vi "Ball Shooter Tasks.vi"(0 "Ball Shooter Task Parameters":T1) -> ()   [LabVIEW 2015]
uses:
  <vilib>/Rock Robotics/WPI/Relay/WPI_RelayValue.ctl
  Robot Global Data.vi
  <vilib>/Rock Robotics/Network Tables/NT Write Number.vi
  <vilib>/Rock Robotics/WPI/Utilities/WPI_GetSetVariantRefNum.vi
  <vilib>/Rock Robotics/Network Tables/NT Read Boolean.vi
  <vilib>/Rock Robotics/WPI/RobotDrive/WPI_RobotDriveArcadeDrive_Standard(NoSaturation).vi
  <vilib>/Rock Robotics/Network Tables/NT Write Numeric Array.vi
  <vilib>/Rock Robotics/Network Tables/NT Read Number.vi
panel:
  out "Shooter Lift Motor":dbl
  out "Drive Motor Values":dbl[](array[numeric])
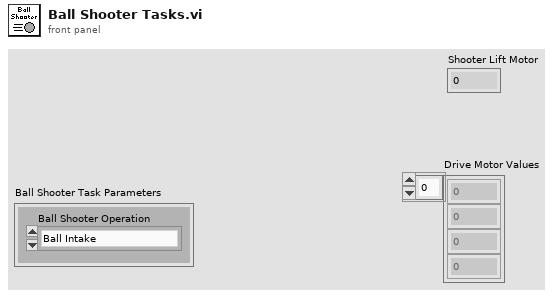
[diagram p1: front panel]
types:
  T1 = cluster{"Ball Shooter Operation":enum16{"Ball Intake", "Fire Ball Shooter", "Aim Ball Shooter"}}
  T2 = typedef "WPI_RelayValue.ctl" = enum16{"Off", "On", "Forward", "Reverse"}
  T3 = enum16{"Ball Intake", "Fire Ball Shooter", "Aim Ball Shooter"}
  T4 = typedef "WPI_MotorControlDeviceRef.ctl" = cluster{"DeviceStatus":errorcluster, "Type":T5, "PWM":cluster{"PWM Channel":T6, "DeadBand":T7}, "CAN":cluster{"Device Number":u8, "Control Mode":T8, "Semaphore":T9, "Max Vout":dbl, "TalonSRX Control Mode":T10}, "Invert":bool}
  T5 = typedef "WPI_MotorControlType.ctl" = enum16{"PWM", "CAN", "CANTalonSRX"}
  T6 = typedef "FPGA_DIOPWMChannel.ctl" = enum8{"PWM 0", "PWM 1", "PWM 2", "PWM 3", "PWM 4", "PWM 5", "PWM 6", "PWM 7", "PWM 8", "PWM 9", "PWM MXP 0", "PWM MXP 1", "PWM MXP 2", "PWM MXP 3", "PWM MXP 4", "PWM MXP 5", "PWM MXP 6", "PWM MXP 7", "PWM MXP 8", "PWM MXP 9", "Invalid"}
  T7 = typedef "WPI_PWMDeadband.ctl" = cluster{"Name":string, "maxPositivePwm":i32, "minPositivePwm":i32, "centerPwm":i32, "maxNegativePwm":i32, "minNegativePwm":i32, "angularRange":u16}
  T8 = typedef "WPI_CANJaguar_ControlMode.ctl" = enum8{"Percent VBus", "Current", "Speed", "Position", "Voltage"}
  T9 = typedef "Semaphore RefNum" = refnum<k1>
  T10 = typedef "WPI_CANTalonSRX_APIControlMode.ctl" = enum8{"Percent VBus", "Speed", "Position", "Slave", "Unchanged / Invalid", "Voltage Compensation", "Current", "Motion Profile"}
  T11 = typedef "WPI_RelayDevRef.ctl" = cluster{"DevStatus":errorcluster, "Relay Channel":T12, "Relay Direction":T13}
  T12 = typedef "FPGA_DIORelayChannel.ctl" = enum8{"Relay 0", "Relay 1", "Relay 2", "Relay 3", "Invalid"}
  T13 = typedef "WPI_RelayDirection.ctl" = enum16{"Both directions", "Forward only", "Reverse only"}
  T14 = typedef "WPI_RobotDriveDevRef.ctl" = cluster{"DevStatus":errorcluster, "Motors[]":T4[], "Square Inputs":bool, "Max Output":dbl}
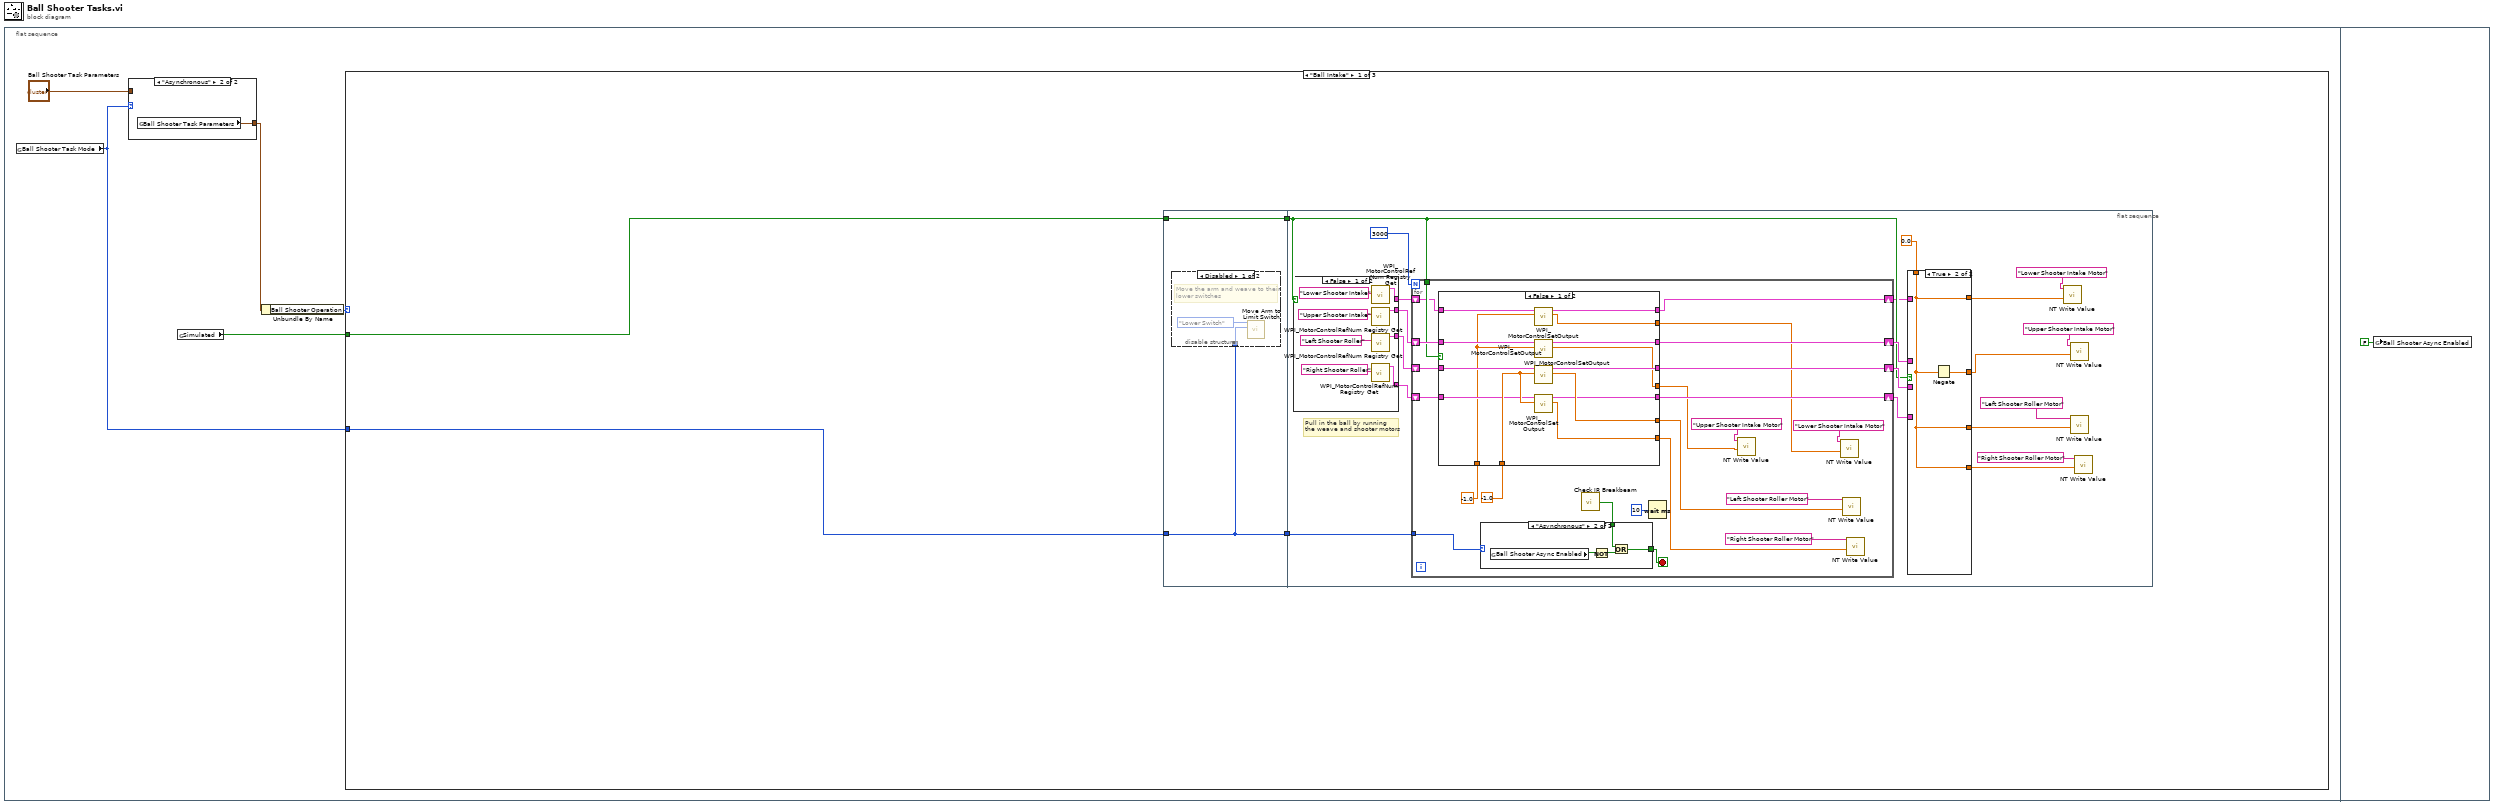
[diagram p0: block diagram]
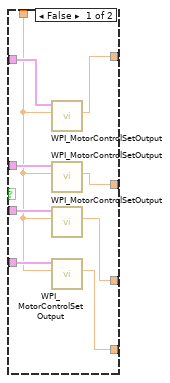
[diagram p4: hidden frame]
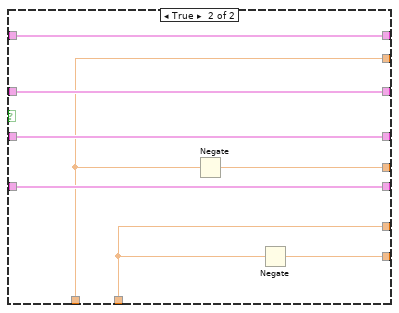
[diagram p5: hidden frame]
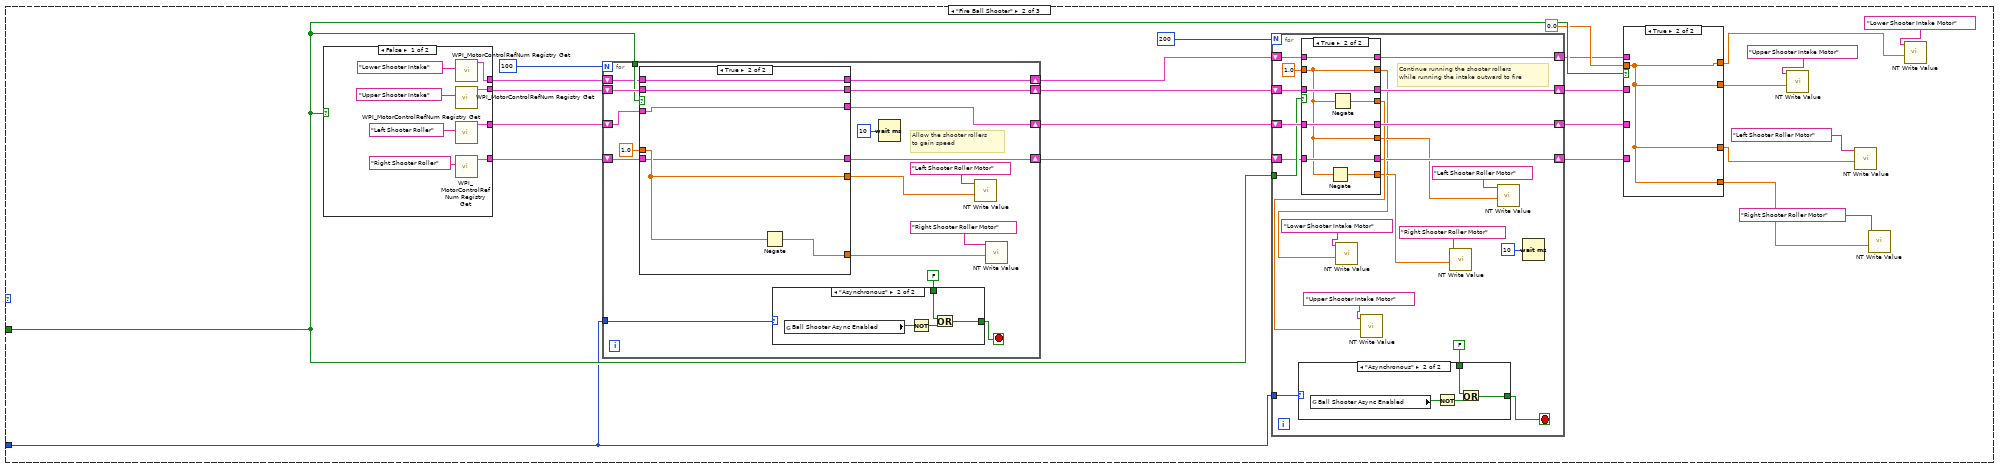
[diagram p7: hidden frame]
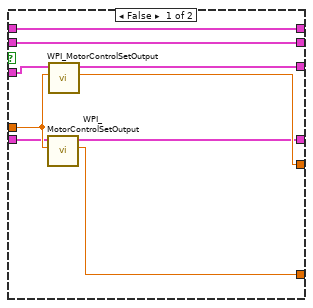
[diagram p8: hidden frame]
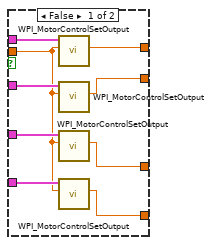
[diagram p10: hidden frame]
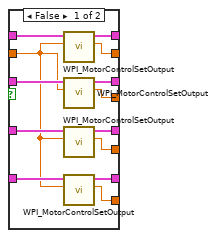
[diagram p12: hidden frame]
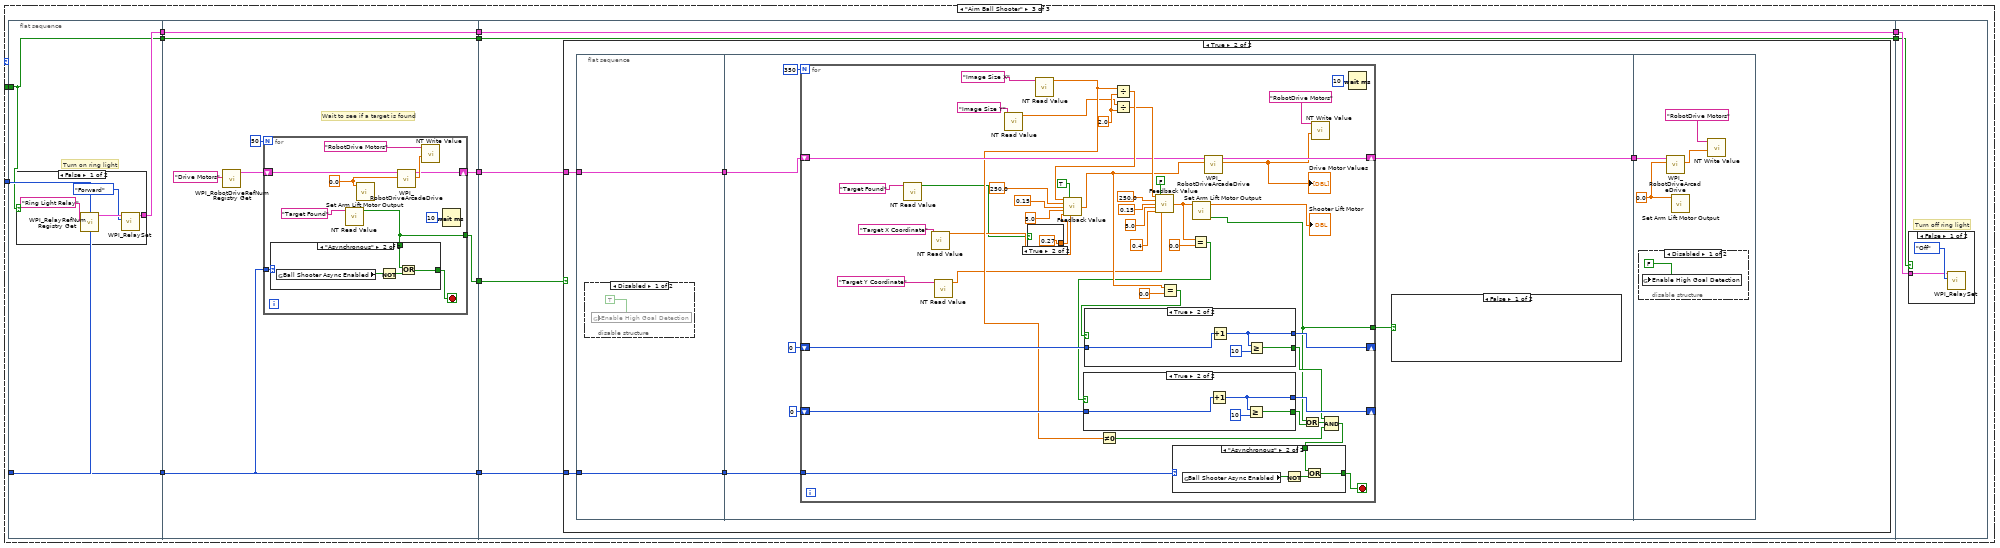
[diagram p14: hidden frame]
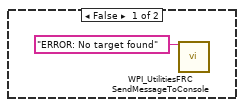
[diagram p17: hidden frame]
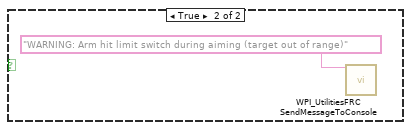
[diagram p19: hidden frame]
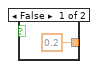
[diagram p20: hidden frame]
diagram:
  n1 = flat-sequence {
    frame #0 {
      n2 = global read "Robot Global Data.vi" "Ball Shooter Task Mode"() -> (w3:enum16{"Synchronous", "Asynchronous"})
      n3 = case shown="\"Asynchronous\"" w3 {
        tunnel: [w370 w371] -> w5
        tunnel: "Ball Shooter Task Parameters" -> [w370 _]
        frame "Synchronous" {
        }
        frame "Asynchronous" {
          n4 = global read "Robot Global Data.vi" "Ball Shooter Task Parameters"() -> (w371:T1)
        }
      }
      n5 = global read "Robot Global Data.vi" "Simulated"() -> (w1:bool)
      n6 = Unbundle By Name(w5) -> ("Ball Shooter Operation"=w4:T3)
      n7 = case shown="\"Ball Intake\"" w4 {
        tunnel: w3 -> [w8 w118 w242]
        tunnel: w1 -> [w9 w119 w235]
        frame "Ball Intake" {
          n8 = flat-sequence {
            tunnel: w8 -> [w10]
            tunnel: w9 -> [w11]
            tunnel: [w11] -> w7
            tunnel: [w10] -> w6
            tunnel: w7 -> [w27]
            tunnel: w6 -> [w30]
            frame #0 {
              n9 = disable-structure shown="Disabled" {
                disable-tunnel: w10 -> [w12 _]
                frame Disabled {
                  # "Move the arm and weave to their\nlower switches"
                  n10 = call "Move Arm to Limit Switch.vi"("Call Mode"=w12, "Switch"=enum16{"Lower Switch", "Upper Switch"}."Lower Switch") -> ()  [unwired: 10 in]
                }
                frame Enabled {
                }
              }
            }
            frame #1 {
              # "Pull in the ball by running\nthe weave and shooter motors"
              n11 = case shown="False" w27 {
                tunnel: [w41 _] -> w29
                tunnel: [w39 _] -> w28
                tunnel: [w36 _] -> w26
                tunnel: [w34 _] -> w19
                frame False {
                  n12 = call <vilib>:"WPI_MotorControlRefNum Registry Get.vi"("refnum name"="Upper Shooter Intake") -> ("MotorControlDevRef"=w39:T4)  [unwired: 9 in, 1 out]
                  n13 = call <vilib>:"WPI_MotorControlRefNum Registry Get.vi"("refnum name"="Left Shooter Roller") -> ("MotorControlDevRef"=w41:T4)  [unwired: 9 in, 1 out]
                  n14 = call <vilib>:"WPI_MotorControlRefNum Registry Get.vi"("refnum name"="Right Shooter Roller") -> ("MotorControlDevRef"=w36:T4)  [unwired: 9 in, 1 out]
                  n15 = call <vilib>:"WPI_MotorControlRefNum Registry Get.vi"("refnum name"="Lower Shooter Intake") -> ("MotorControlDevRef"=w34:T4)  [unwired: 9 in, 1 out]
                }
                frame True {
                }
              }
              n16 = for {
                N: 3000 -> [_]
                tunnel: w30 -> [w75]
                shift-right: [w71] -> w31
                shift-left: w28 -> [w72]
                shift-right: [w69] -> w32
                shift-left: w29 -> [w70]
                tunnel: w27 -> [w68]
                shift-right: [w60] -> w25
                shift-left: w26 -> [w61]
                shift-right: [w56] -> w18
                shift-left: w19 -> [w57]
                stop <- w74 stop-if-true
                n17 = case shown="False" w68 {
                  tunnel: w72 -> [w89 w97]
                  tunnel: [w88 w97] -> w71
                  tunnel: w70 -> [w87 w96]
                  tunnel: [w86 w96] -> w69
                  tunnel: [w85 w91] -> w54
                  tunnel: [w84 w93] -> w65
                  tunnel: -1.0 -> [w83 w93]
                  tunnel: -1.0 -> [w77 w90]
                  tunnel: w61 -> [w82 w95]
                  tunnel: [w81 w95] -> w60
                  tunnel: [w80 w94] -> w58
                  tunnel: w57 -> [w79 w92]
                  tunnel: [w78 w92] -> w56
                  tunnel: [w76 w90] -> w53
                  frame False {
                    n18 = call <vilib>:"WPI_MotorControlSetOutput.vi"("Output"=w77, "MotorControlDevRef"=w79) -> ("Motor Output"=w76:dbl, "MotorControlDevRef"=w78:T4)  [unwired: 7 in, 1 out]
                    n19 = call <vilib>:"WPI_MotorControlSetOutput.vi"("Output"=w77, "MotorControlDevRef"=w89) -> ("Motor Output"=w85:dbl, "MotorControlDevRef"=w88:T4)  [unwired: 7 in, 1 out]
                    n20 = call <vilib>:"WPI_MotorControlSetOutput.vi"("Output"=w83, "MotorControlDevRef"=w87) -> ("Motor Output"=w84:dbl, "MotorControlDevRef"=w86:T4)  [unwired: 7 in, 1 out]
                    n21 = call <vilib>:"WPI_MotorControlSetOutput.vi"("Output"=w83, "MotorControlDevRef"=w82) -> ("Motor Output"=w80:dbl, "MotorControlDevRef"=w81:T4)  [unwired: 7 in, 1 out]
                  }
                  frame True {
                    n22 = Negate(x=w90) -> (-x=w91:dbl)
                    n23 = Negate(x=w93) -> (-x=w94:dbl)
                  }
                }
                n24 = call "Check IR Breakbeam.vi"() -> ("Beam Broken"=w67:bool)
                n25 = case shown="\"Asynchronous\"" w75 {
                  tunnel: [w98 w100] -> w74
                  tunnel: w67 -> [w98 w99]
                  frame "Synchronous" {
                  }
                  frame "Asynchronous" {
                    n26 = global read "Robot Global Data.vi" "Ball Shooter Async Enabled"() -> (w101:bool)
                    n27 = Not(x=w101) -> (.not. x?=w102:bool)
                    n28 = Or(x=w99, y=w102) -> (x .or. y?=w100:bool)
                  }
                }
                n29 = Wait (ms)(milliseconds to wait=u32 10) -> ()  [unwired: 1 out]
                n30 = call-poly <vilib>:"NT Write Value.vi"("Numeric"=w54, "Name"="Upper Shooter Intake Motor" ("refnum name")) -> ()  [unwired: 9 in, 1 out]
                n31 = call-poly <vilib>:"NT Write Value.vi"("Numeric"=w53, "Name"="Lower Shooter Intake Motor" ("refnum name")) -> ()  [unwired: 9 in, 1 out]
                n32 = call-poly <vilib>:"NT Write Value.vi"("Numeric"=w65, "Name"="Left Shooter Roller Motor" ("refnum name")) -> ()  [unwired: 9 in, 1 out]
                n33 = call-poly <vilib>:"NT Write Value.vi"("Numeric"=w58, "Name"="Right Shooter Roller Motor" ("refnum name")) -> ()  [unwired: 9 in, 1 out]
              }
              n34 = case shown="True" w27 {
                tunnel: w32 -> [w50 _]
                tunnel: w31 -> [w49 _]
                tunnel: w25 -> [w48 _]
                tunnel: [w47 w52] -> w14
                tunnel: [w46 w51] -> w22
                tunnel: [w45 w51] -> w21
                tunnel: 0.0 -> [w43 w51]
                tunnel: w18 -> [w44 _]
                tunnel: [w42 w51] -> w15
                frame False {
                  n35 = call <vilib>:"WPI_MotorControlSetOutput.vi"("Output"=w43, "MotorControlDevRef"=w44) -> ("Motor Output"=w42:dbl)  [unwired: 7 in, 2 out]
                  n36 = call <vilib>:"WPI_MotorControlSetOutput.vi"("Output"=w43, "MotorControlDevRef"=w49) -> ("Motor Output"=w47:dbl)  [unwired: 7 in, 2 out]
                  n37 = call <vilib>:"WPI_MotorControlSetOutput.vi"("Output"=w43, "MotorControlDevRef"=w50) -> ("Motor Output"=w46:dbl)  [unwired: 7 in, 2 out]
                  n38 = call <vilib>:"WPI_MotorControlSetOutput.vi"("Output"=w43, "MotorControlDevRef"=w48) -> ("Motor Output"=w45:dbl)  [unwired: 7 in, 2 out]
                }
                frame True {
                  n39 = Negate(x=w51) -> (-x=w52:dbl)
                }
              }
              n40 = call-poly <vilib>:"NT Write Value.vi"("Numeric"=w15, "Name"="Lower Shooter Intake Motor" ("refnum name")) -> ()  [unwired: 9 in, 1 out]
              n41 = call-poly <vilib>:"NT Write Value.vi"("Numeric"=w14, "Name"="Upper Shooter Intake Motor" ("refnum name")) -> ()  [unwired: 9 in, 1 out]
              n42 = call-poly <vilib>:"NT Write Value.vi"("Numeric"=w22, "Name"="Left Shooter Roller Motor" ("refnum name")) -> ()  [unwired: 9 in, 1 out]
              n43 = call-poly <vilib>:"NT Write Value.vi"("Numeric"=w21, "Name"="Right Shooter Roller Motor" ("refnum name")) -> ()  [unwired: 9 in, 1 out]
            }
          }
        }
        frame "Fire Ball Shooter" {
          n44 = case shown="False" w119 {
            tunnel: [w182 _] -> w123
            tunnel: [w179 _] -> w122
            tunnel: [w178 _] -> w114
            tunnel: [w176 _] -> w107
            frame False {
              n45 = call <vilib>:"WPI_MotorControlRefNum Registry Get.vi"("refnum name"="Upper Shooter Intake") -> ("MotorControlDevRef"=w182:T4)  [unwired: 9 in, 1 out]
              n46 = call <vilib>:"WPI_MotorControlRefNum Registry Get.vi"("refnum name"="Left Shooter Roller") -> ("MotorControlDevRef"=w179:T4)  [unwired: 9 in, 1 out]
              n47 = call <vilib>:"WPI_MotorControlRefNum Registry Get.vi"("refnum name"="Right Shooter Roller") -> ("MotorControlDevRef"=w178:T4)  [unwired: 9 in, 1 out]
              n48 = call <vilib>:"WPI_MotorControlRefNum Registry Get.vi"("refnum name"="Lower Shooter Intake") -> ("MotorControlDevRef"=w176:T4)  [unwired: 9 in, 1 out]
            }
            frame True {
            }
          }
          n49 = for {
            N: 100 -> [_]
            shift-right: [w139] -> w121
            shift-left: w122 -> [w140]
            shift-right: [w142] -> w120
            shift-left: w123 -> [w141]
            tunnel: w119 -> [w138]
            tunnel: w118 -> [w137]
            shift-right: [w130] -> w113
            shift-left: w114 -> [w131]
            shift-right: [w128] -> w106
            shift-left: w107 -> [w129]
            stop <- w144 stop-if-true
            # "Allow the shooter rollers\nto gain speed"
            n50 = case shown="True" w138 {
              tunnel: [w154 w160] -> w142
              tunnel: w141 -> [w154 w160]
              tunnel: w140 -> [w153 w159]
              tunnel: [w152 w159] -> w139
              tunnel: 1.0 ("Output") -> [w151 w157]
              tunnel: [w150 w157] -> w133
              tunnel: [w149 w158] -> w132
              tunnel: w131 -> [w148 w156]
              tunnel: [w147 w156] -> w130
              tunnel: w129 -> [w146 w155]
              tunnel: [w146 w155] -> w128
              frame False {
                n51 = call <vilib>:"WPI_MotorControlSetOutput.vi"("Output"=w151, "MotorControlDevRef"=w148) -> ("Motor Output"=w149:dbl, "MotorControlDevRef"=w147:T4)  [unwired: 7 in, 1 out]
                n52 = call <vilib>:"WPI_MotorControlSetOutput.vi"("Output"=w151, "MotorControlDevRef"=w153) -> ("Motor Output"=w150:dbl, "MotorControlDevRef"=w152:T4)  [unwired: 7 in, 1 out]
              }
              frame True {
                n53 = Negate(x=w157) -> (-x=w158:dbl)
              }
            }
            n54 = case shown="\"Asynchronous\"" w137 {
              tunnel: FALSE -> [w161 w163]
              tunnel: [w161 w162] -> w144
              frame "Synchronous" {
              }
              frame "Asynchronous" {
                n55 = global read "Robot Global Data.vi" "Ball Shooter Async Enabled"() -> (w164:bool)
                n56 = Not(x=w164) -> (.not. x?=w165:bool)
                n57 = Or(x=w163, y=w165) -> (x .or. y?=w162:bool)
              }
            }
            n58 = Wait (ms)(milliseconds to wait=u32 10) -> ()  [unwired: 1 out]
            n59 = call-poly <vilib>:"NT Write Value.vi"("Numeric"=w133, "Name"="Left Shooter Roller Motor" ("refnum name")) -> ()  [unwired: 9 in, 1 out]
            n60 = call-poly <vilib>:"NT Write Value.vi"("Numeric"=w132, "Name"="Right Shooter Roller Motor" ("refnum name")) -> ()  [unwired: 9 in, 1 out]
          }
          n61 = for {
            N: 200 -> [_]
            shift-right: [w202] -> w127
            shift-left: w120 -> [w204]
            shift-right: [w201] -> w126
            shift-left: w121 -> [w203]
            tunnel: w118 -> [w199]
            tunnel: w119 -> [w197]
            shift-right: [w190] -> w112
            shift-left: w113 -> [w191]
            shift-right: [w186] -> w105
            shift-left: w106 -> [w187]
            stop <- w205 stop-if-true
            # "Continue running the shooter rollers\nwhile running the intake outward to fire"
            n62 = case shown="\"Asynchronous\"" w199 {
              tunnel: FALSE -> [w226 w228]
              tunnel: [w226 w227] -> w205
              frame "Synchronous" {
              }
              frame "Asynchronous" {
                n63 = global read "Robot Global Data.vi" "Ball Shooter Async Enabled"() -> (w229:bool)
                n64 = Not(x=w229) -> (.not. x?=w230:bool)
                n65 = Or(x=w228, y=w230) -> (x .or. y?=w227:bool)
              }
            }
            n66 = case shown="True" w197 {
              tunnel: w204 -> [w218 w225]
              tunnel: w203 -> [w217 w224]
              tunnel: [w216 w225] -> w202
              tunnel: [w215 w224] -> w201
              tunnel: [w214 w220] -> w195
              tunnel: [w213 w219] -> w189
              tunnel: 1.0 -> [w209 w219]
              tunnel: w191 -> [w212 w223]
              tunnel: [w211 w223] -> w190
              tunnel: [w210 w222] -> w188
              tunnel: w187 -> [w208 w221]
              tunnel: [w207 w221] -> w186
              tunnel: [w206 w219] -> w184
              frame False {
                n67 = call <vilib>:"WPI_MotorControlSetOutput.vi"("Output"=w209, "MotorControlDevRef"=w208) -> ("Motor Output"=w206:dbl, "MotorControlDevRef"=w207:T4)  [unwired: 7 in, 1 out]
                n68 = call <vilib>:"WPI_MotorControlSetOutput.vi"("Output"=w209, "MotorControlDevRef"=w218) -> ("Motor Output"=w214:dbl, "MotorControlDevRef"=w216:T4)  [unwired: 7 in, 1 out]
                n69 = call <vilib>:"WPI_MotorControlSetOutput.vi"("Output"=w209, "MotorControlDevRef"=w217) -> ("Motor Output"=w213:dbl, "MotorControlDevRef"=w215:T4)  [unwired: 7 in, 1 out]
                n70 = call <vilib>:"WPI_MotorControlSetOutput.vi"("Output"=w209, "MotorControlDevRef"=w212) -> ("Motor Output"=w210:dbl, "MotorControlDevRef"=w211:T4)  [unwired: 7 in, 1 out]
              }
              frame True {
                n71 = Negate(x=w219) -> (-x=w222:dbl)
                n72 = Negate(x=w219) -> (-x=w220:dbl)
              }
            }
            n73 = call-poly <vilib>:"NT Write Value.vi"("Numeric"=w184, "Name"="Lower Shooter Intake Motor" ("refnum name")) -> ()  [unwired: 9 in, 1 out]
            n74 = call-poly <vilib>:"NT Write Value.vi"("Numeric"=w195, "Name"="Upper Shooter Intake Motor" ("refnum name")) -> ()  [unwired: 9 in, 1 out]
            n75 = call-poly <vilib>:"NT Write Value.vi"("Numeric"=w188, "Name"="Right Shooter Roller Motor" ("refnum name")) -> ()  [unwired: 9 in, 1 out]
            n76 = call-poly <vilib>:"NT Write Value.vi"("Numeric"=w189, "Name"="Left Shooter Roller Motor" ("refnum name")) -> ()  [unwired: 9 in, 1 out]
            n77 = Wait (ms)(milliseconds to wait=u32 10) -> ()  [unwired: 1 out]
          }
          n78 = case shown="True" w119 {
            tunnel: w127 -> [w174 _]
            tunnel: w126 -> [w173 _]
            tunnel: 0.0 -> [w167 w175]
            tunnel: [w172 w175] -> w115
            tunnel: [w171 w175] -> w109
            tunnel: w112 -> [w170 _]
            tunnel: [w169 w175] -> w108
            tunnel: w105 -> [w168 _]
            tunnel: [w166 w175] -> w103
            frame False {
              n79 = call <vilib>:"WPI_MotorControlSetOutput.vi"("Output"=w167, "MotorControlDevRef"=w168) -> ("Motor Output"=w166:dbl)  [unwired: 7 in, 2 out]
              n80 = call <vilib>:"WPI_MotorControlSetOutput.vi"("Output"=w167, "MotorControlDevRef"=w174) -> ("Motor Output"=w172:dbl)  [unwired: 7 in, 2 out]
              n81 = call <vilib>:"WPI_MotorControlSetOutput.vi"("Output"=w167, "MotorControlDevRef"=w173) -> ("Motor Output"=w171:dbl)  [unwired: 7 in, 2 out]
              n82 = call <vilib>:"WPI_MotorControlSetOutput.vi"("Output"=w167, "MotorControlDevRef"=w170) -> ("Motor Output"=w169:dbl)  [unwired: 7 in, 2 out]
            }
            frame True {
            }
          }
          n83 = call-poly <vilib>:"NT Write Value.vi"("Numeric"=w115, "Name"="Upper Shooter Intake Motor" ("refnum name")) -> ()  [unwired: 9 in, 1 out]
          n84 = call-poly <vilib>:"NT Write Value.vi"("Numeric"=w109, "Name"="Left Shooter Roller Motor" ("refnum name")) -> ()  [unwired: 9 in, 1 out]
          n85 = call-poly <vilib>:"NT Write Value.vi"("Numeric"=w108, "Name"="Right Shooter Roller Motor" ("refnum name")) -> ()  [unwired: 9 in, 1 out]
          n86 = call-poly <vilib>:"NT Write Value.vi"("Numeric"=w103, "Name"="Lower Shooter Intake Motor" ("refnum name")) -> ()  [unwired: 9 in, 1 out]
        }
        frame "Aim Ball Shooter" {
          n87 = flat-sequence {
            tunnel: w242 -> [w245]
            tunnel: [w245] -> w241
            tunnel: [w244] -> w236
            tunnel: w235 -> [w243]
            tunnel: [w243] -> w232
            tunnel: w241 -> [w255]
            tunnel: [w255] -> w240
            tunnel: [w256] -> w239
            tunnel: [w254] -> w237
            tunnel: w236 -> [w254]
            tunnel: [w253] -> w233
            tunnel: w232 -> [w253]
            tunnel: [w250] -> w231
            tunnel: w240 -> [w277]
            tunnel: w239 -> [w276]
            tunnel: [w275] -> w238
            tunnel: w237 -> [w275]
            tunnel: [w274] -> w234
            tunnel: w233 -> [w274]
            tunnel: w231 -> [w273]
            tunnel: w238 -> [w367]
            tunnel: w234 -> [w366]
            frame #0 {
              # "Turn on ring light"
              n88 = case shown="False" w243 {
                tunnel: [w246 _] -> w244
                frame False {
                  n89 = call <vilib>:"WPI_RelayRefNum Registry Get.vi"("refnum name"="Ring Light Relay") -> ("RelayDevRef"=w248:T11)  [unwired: 9 in, 1 out]
                  n90 = call <vilib>:"WPI_RelaySet.vi"("RelayValue"=WPI_RelayValue."Forward", "RelayDevRef"=w248) -> ("RelayDevRef"=w246:T11)  [unwired: 8 in, 1 out]
                }
                frame True {
                }
              }
            }
            frame #1 {
              # "Wait to see if a target is found"
              n91 = call <vilib>:"WPI_RobotDriveRefNum Registry Get.vi"("refnum name"="Drive Motors") -> ("RobotDriveDevRef"=w251:T14)  [unwired: 9 in, 1 out]
              n92 = for {
                N: 50 -> [_]
                tunnel: [w264] -> w256
                tunnel: w255 -> [w263]
                shift-right: [w258] -> w250
                shift-left: w251 -> [w259]
                stop <- w266 stop-if-true
                w260 = 0.0
                n93 = call-poly <vilib>:"NT Read Value.vi"("Name"="Target Found") -> ("Boolean"=w264:bool)  [unwired: 9 in, 1 out]
                n94 = case shown="\"Asynchronous\"" w263 {
                  tunnel: [w268 w270] -> w266
                  tunnel: w264 -> [w268 w269]
                  frame "Synchronous" {
                  }
                  frame "Asynchronous" {
                    n95 = global read "Robot Global Data.vi" "Ball Shooter Async Enabled"() -> (w271:bool)
                    n96 = Not(x=w271) -> (.not. x?=w272:bool)
                    n97 = Or(x=w269, y=w272) -> (x .or. y?=w270:bool)
                  }
                }
                n98 = call "Set Arm Lift Motor Output.vi"("Output"=w260) -> ()  [unwired: 7 in, 4 out]
                n99 = call-poly <vilib>:"WPI_RobotDriveArcadeDrive.vi"("X axis value"=w260, "RobotDriveDevRef"=w259) -> ("Motor Values"=w262:dbl[], "RobotDriveDevRef"=w258:T14)  [unwired: 7 in, 1 out]
                n100 = call-poly <vilib>:"NT Write Value.vi"("Numeric Array"=w262, "Name"="RobotDrive Motors") -> ()  [unwired: 9 in, 1 out]
                n101 = Wait (ms)(milliseconds to wait=u32 10) -> ()  [unwired: 1 out]
              }
            }
            frame #2 {
              n102 = case shown="True" w276 {
                tunnel: w277 -> [_ w281]
                tunnel: w273 -> [_ w279]
                frame False {
                  n103 = call <vilib>:"WPI_UtilitiesFRC SendMessageToConsole.vi"("Message"="ERROR: No target found") -> ()  [unwired: 14 in, 1 out]
                }
                frame True {
                  n104 = flat-sequence {
                    tunnel: w281 -> [w285]
                    tunnel: [w285] -> w283
                    tunnel: [w284] -> w280
                    tunnel: w279 -> [w284]
                    tunnel: w283 -> [w292]
                    tunnel: [w288] -> w282
                    tunnel: w280 -> [w287]
                    tunnel: w282 -> [w362]
                    frame #0 {
                      n105 = disable-structure shown="Disabled" {
                        frame Disabled {
                          n106 = global write "Robot Global Data.vi" "Enable High Goal Detection"(TRUE ("Enable Vision")) -> ()
                        }
                        frame Enabled {
                        }
                      }
                    }
                    frame #1 {
                      n107 = for {
                        N: 350 -> [_]
                        shift-right: [w327] -> w288
                        shift-left: w287 -> [w328]
                        tunnel: w292 -> [w324]
                        shift-right: [w320] -> _
                        shift-left: 0 -> [w321]
                        shift-right: [w318] -> _
                        shift-left: 0 -> [w319]
                        tunnel: [w307] -> w289
                        stop <- w325 stop-if-true
                        w336 = 2.0
                        n108 = call-poly <vilib>:"NT Read Value.vi"("Name"="Target Found") -> ("Boolean"=w296:bool)  [unwired: 9 in, 1 out]
                        n109 = call-poly <vilib>:"NT Read Value.vi"("Name"="Target X Coordinate") -> ("Numeric"=w299:dbl)  [unwired: 9 in, 1 out]
                        n110 = call-poly <vilib>:"NT Read Value.vi"("Name"="Target Y Coordinate") -> ("Numeric"=w298:dbl)  [unwired: 9 in, 1 out]
                        n111 = call-poly <vilib>:"NT Read Value.vi"("Name"="Image Size Y") -> ("Numeric"=w302:dbl)  [unwired: 9 in, 1 out]
                        n112 = case shown="True" w296 {
                          tunnel: [0.2 ("Maximum Amplitude") 0.27 ("Maximum Amplitude")] -> w340
                          frame False {
                          }
                          frame True {
                          }
                        }
                        n113 = call-poly <vilib>:"NT Read Value.vi"("Name"="Image Size X") -> ("Numeric"=w303:dbl)  [unwired: 9 in, 1 out]
                        n114 = Not Equal To 0?(x=w303) -> (x != 0?=w306:bool)
                        n115 = Divide(x=w303, y=w336) -> (x/y=w335:dbl)
                        n116 = call "Feedback Value.vi"("Set Point"=w335, "Invert Rotation"=TRUE, "Divisor"=250.0, "Addend"=0.15, "Deadband"=5.0, "Maximum Amplitude"=w340, "Current Value"=w299) -> ("Rotation"=w312:dbl)  [unwired: 8 in]
                        n117 = Divide(x=w302, y=w336) -> (x/y=w334:dbl)
                        n118 = call "Feedback Value.vi"("Set Point"=w334, "Invert Rotation"=FALSE, "Divisor"=250.0, "Addend"=0.15, "Deadband"=5.0, "Maximum Amplitude"=0.4, "Current Value"=w298) -> ("Rotation"=w315:dbl)  [unwired: 8 in]
                        n119 = Equal?(x=w312, y=0.0) -> (x = y?=w311:bool)
                        n120 = case shown="True" w311 {
                          tunnel: [0 w354] -> w320
                          tunnel: w321 -> [_ w355]
                          tunnel: [FALSE w352] -> w317
                          frame False {
                          }
                          frame True {
                            n121 = Increment(x=w355) -> (x+1=w354:i32)
                            n122 = Greater Or Equal?(x=w354, y=10) -> (x >= y?=w352:bool)
                          }
                        }
                        n123 = Equal?(x=w315, y=0.0) -> (x = y?=w310:bool)
                        n124 = case shown="True" w310 {
                          tunnel: [0 w348] -> w318
                          tunnel: w319 -> [_ w349]
                          tunnel: [FALSE w346] -> w308
                          frame False {
                          }
                          frame True {
                            n125 = Increment(x=w349) -> (x+1=w348:i32)
                            n126 = Greater Or Equal?(x=w348, y=10) -> (x >= y?=w346:bool)
                          }
                        }
                        n127 = call "Set Arm Lift Motor Output.vi"("Output"=w315) -> ("Switch Stop"=w307:bool, "Shooter Lift Motor"=→"Shooter Lift Motor":dbl)  [unwired: 7 in, 2 out]
                        n128 = call-poly <vilib>:"WPI_RobotDriveArcadeDrive.vi"("X axis value"=w312, "RobotDriveDevRef"=w328) -> ("Motor Values"=w322:dbl[], "RobotDriveDevRef"=w327:T14)  [unwired: 7 in, 1 out]
                        "Drive Motor Values" <- w322
                        n129 = Or(x=w307, y=w308) -> (x .or. y?=w309:bool)
                        n130 = call-poly <vilib>:"NT Write Value.vi"("Numeric Array"=w322, "Name"="RobotDrive Motors") -> ()  [unwired: 9 in, 1 out]
                        n131 = Compound Arithmetic op=AND(w317, w309, w306) -> (w316:bool)
                        n132 = case shown="\"Asynchronous\"" w324 {
                          tunnel: [w356 w358] -> w325
                          tunnel: w316 -> [w356 w357]
                          frame "Synchronous" {
                          }
                          frame "Asynchronous" {
                            n133 = global read "Robot Global Data.vi" "Ball Shooter Async Enabled"() -> (w359:bool)
                            n134 = Not(x=w359) -> (.not. x?=w360:bool)
                            n135 = Or(x=w357, y=w360) -> (x .or. y?=w358:bool)
                          }
                        }
                        n136 = Wait (ms)(milliseconds to wait=u32 10) -> ()  [unwired: 1 out]
                      }
                      n137 = case shown="False" w289 {
                        frame False {
                        }
                        frame True {
                          n138 = call <vilib>:"WPI_UtilitiesFRC SendMessageToConsole.vi"("Message"="WARNING: Arm hit limit switch during aiming (target out of range)") -> ()  [unwired: 14 in, 1 out]
                        }
                      }
                    }
                    frame #2 {
                      w361 = 0.0
                      n139 = disable-structure shown="Disabled" {
                        frame Disabled {
                          n140 = global write "Robot Global Data.vi" "Enable High Goal Detection"(FALSE ("Enable Vision")) -> ()
                        }
                        frame Enabled {
                        }
                      }
                      n141 = call-poly <vilib>:"WPI_RobotDriveArcadeDrive.vi"("X axis value"=w361, "RobotDriveDevRef"=w362) -> ("Motor Values"=w364:dbl[])  [unwired: 7 in, 2 out]
                      n142 = call "Set Arm Lift Motor Output.vi"("Output"=w361) -> ()  [unwired: 7 in, 4 out]
                      n143 = call-poly <vilib>:"NT Write Value.vi"("Numeric Array"=w364, "Name"="RobotDrive Motors") -> ()  [unwired: 9 in, 1 out]
                    }
                  }
                }
              }
            }
            frame #3 {
              # "Turn off ring light"
              n144 = case shown="False" w366 {
                tunnel: w367 -> [w368 _]
                frame False {
                  n145 = call <vilib>:"WPI_RelaySet.vi"("RelayValue"=WPI_RelayValue."Off", "RelayDevRef"=w368) -> ()  [unwired: 8 in, 2 out]
                }
                frame True {
                }
              }
            }
          }
        }
      }
    }
    frame #1 {
      n146 = global write "Robot Global Data.vi" "Ball Shooter Async Enabled"(FALSE ("Ball Shooter Async Enabled")) -> ()
    }
  }
